vi "Actor Core.vi"(8 "error in":errorcluster, 11 "Controller in":refnum<class "Controller.lvclass">) -> (0 "error out":errorcluster, 3 "Actor out":refnum<class "Actor.lvclass">)   [LabVIEW 2011, in "Controller.lvclass"]
doc: "(<B>Filename</B>: Actor Framework.lvlib:Actor.lvclass:Actor Core.vi)\n\nReceives messages to the actor, reacts to them, and initiates any error handling that may shut the actor down.\n\nDescendant classes may override this VI to append parallel tasks for the actor to complete while it handles messages. Overrides use the Call Parent Method node."
uses:
  Controller.lvclass
  <userlib>/_Frameworks/ActorFramework/Actor/Actor.lvclass
  Controls/UI Elements.ctl
  Controller.lvclass/Controller.ctl
  <userlib>/_Frameworks/ActorFramework/Actor/Actor.lvclass/Actor.ctl
  <userlib>/_Frameworks/ActorFramework/Message Enqueuer/Message Enqueuer.lvclass/Message Enqueuer.ctl
  <userlib>/_Frameworks/ActorFramework/Message Enqueuer/Init from Existing Queue.vi
  <userlib>/_Frameworks/ActorFramework/Message Enqueuer/Enqueue.vi
  <userlib>/_Frameworks/ActorFramework/Message Priority Queue/Priority Enqueue.vi
  <userlib>/_Frameworks/ActorFramework/Message Enqueuer/Message Enqueuer.lvclass
  <userlib>/_Frameworks/ActorFramework/Stop Msg/Stop Msg.lvclass
panel:
  in  "Stop Button":bool
  out "Pulse":dbl(graph)
  out "EDR":dbl(graph)
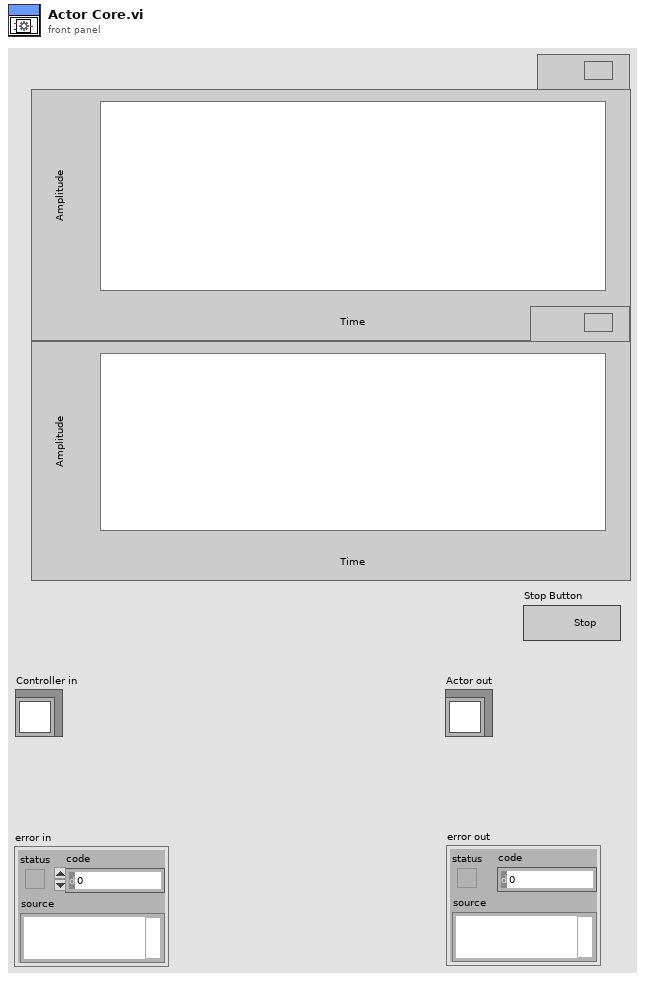
[diagram p1: front panel]
types:
  T1 = typedef "Controller.lvclass/UI Elements.ctl" = cluster{"Pulse":refnum<vi>, "EDR":refnum<vi>}
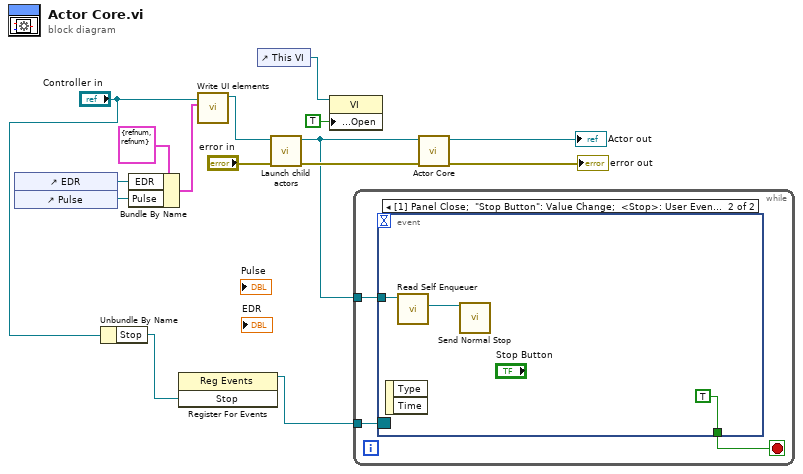
[diagram p0: block diagram]
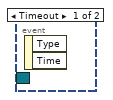
[diagram p2: hidden frame]
diagram:
  n1 = control-ref of="EDR"() -> (w8:refnum<vi>)
  n2 = control-ref of="Pulse"() -> (w7:refnum<vi>)
  n3 = Unbundle By Name("Controller in") -> ("Stop"=w2:refnum<user-event>)
  n4 = Bundle By Name(cluster=T1 {"Pulse"=refnum, "EDR"=refnum} ("UI elements"), "EDR"=w8, "Pulse"=w7) -> (w6:T1)
  n5 = register-events(w2) -> (reference out=w1:refnum<event-registration>)  [unwired: 2 in, 1 out]
  n6 = call "Write UI elements.vi"("UI elements"=w6, "Controller in"="Controller in") -> ("Controller out"=w4:refnum<class "Controller.lvclass">)  [unwired: 9 in]
  n7 = control-ref of="This VI"() -> (w11:refnum<vi>)
  n8 = call-dynamic "Launch child actors.vi"("error in (no error)"="error in", "Controller in"=w4) -> ("error out"=w12:errorcluster, "Controller out"=w5:refnum<class "Controller.lvclass">)  [unwired: 8 in]
  n9 = property class="VI"(reference=w11, "Front Panel.Open"=TRUE ("Front Panel Window:Open")) -> ()  [unwired: 1 in, 2 out]
  n10 = while {
    tunnel: w5 -> [w18]
    tunnel: w1 -> [w16]
    stop <- w17 stop-if-true
    n11 = event shown="[1] Panel Close;  \"Stop Button\": Value Change;  <Stop>: User Event" {
      selector: w16 -> [_ _]
      dyn-events: _ -> [_ _]
      timeout: _ -> [_ _]
      tunnel: w18 -> [_ w20]
      tunnel: [_ TRUE] -> w17
      event Timeout {
        n12 = event-data() -> ()  [unwired: 1 in, 2 out]
      }
      event Panel Close; "Stop Button": Value Change; User Event {
        n13 = event-data() -> ()  [unwired: 1 in, 2 out]
        n14 = call <userlib>:"Read Self Enqueuer.vi"("Actor"=w20) -> ("Self Enqueuer"=w21:refnum<class "Message Enqueuer.lvclass">)  [unwired: 10 in]
        n15 = call <userlib>:"Send Normal Stop.vi"("Message Enqueuer"=w21) -> ()  [unwired: 10 in, 1 out]
      }
    }
  }
  n16 = call-parent "Actor Core.vi"("error in"=w12, "Actor in"=w5) -> ("error out"=→"error out":errorcluster, "Actor out"=→"Actor out":refnum<class "Actor.lvclass">)  [unwired: 8 in]
